vi "Replace Board Pixels.vi"(8 "error in (no error)":errorcluster caption="entrée d'erreur (pas d'erreur)", 9 "New pixels color":u32(colorbox), 10 "Pixels":T1[](array[typedef]), 11 "Game Board en entrée":refnum<class "Game Board.lvclass">) -> (0 "error out":errorcluster caption="sortie d'erreur", 3 "Game Board en sortie":refnum<class "Game Board.lvclass">)   [LabVIEW 2017, in "Game Board.lvclass"]
uses:
  Game Board.lvclass
  Controls/Coordinates.ctl
  Game Board.lvclass/Game Board.ctl
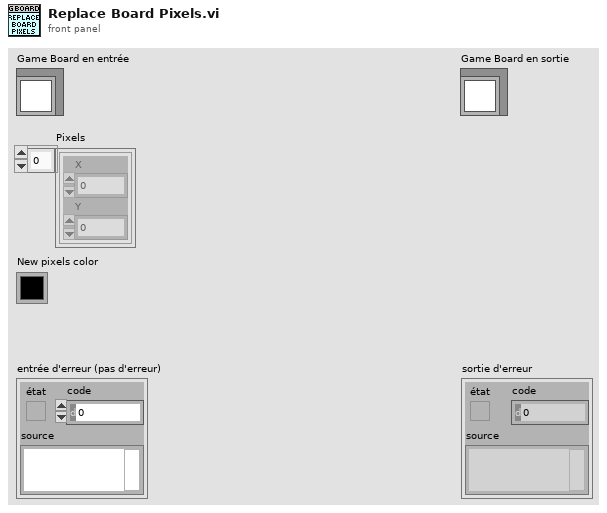
[diagram p1: front panel]
types:
  T1 = typedef "Coordinates.ctl" = cluster{"X":i32, "Y":i32}
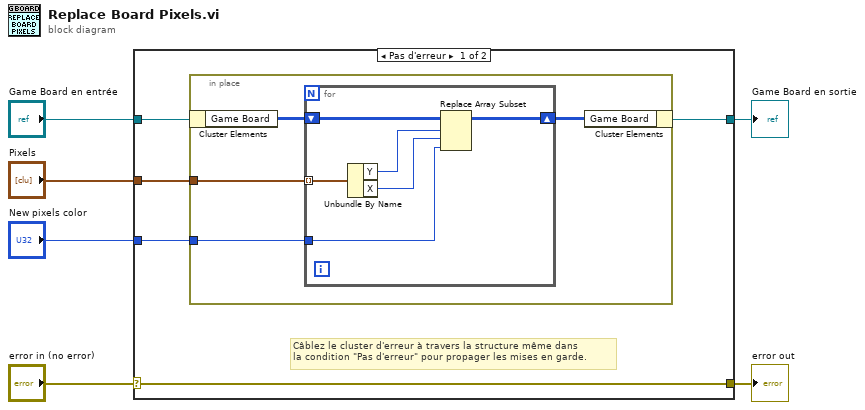
[diagram p0: block diagram]
diagram:
  n1 = case shown="Pas d'erreur" "error in (no error)" {
    selector: "error in (no error)" -> [w11 w23]
    tunnel: [w11 w23] -> w5
    tunnel: [w9 w22] -> w3
    tunnel: "Game Board en entrée" -> [w10 w22]
    tunnel: "Pixels" -> [w8 _]
    tunnel: "New pixels color" -> [w7 _]
    frame No Error {
      # "Câblez le cluster d'erreur à travers la structure même dans\nla condition \"Pas d'erreur\" pour propager les mises en garde."
      n2 = in-place {
        in-place-border: w8 -> [w13]
        in-place-border: w7 -> [w12]
        n3 = in-place-cluster #1(w10) -> ("Game Board"=w15:u32[][])
        n4 = for {
          shift-right: [w20] -> w14
          shift-left: w15 -> [w21]
          tunnel: w13 -> [w19] mode=indexing
          tunnel: w12 -> [w16]
          n5 = Unbundle By Name(w19) -> ("Y"=w18:i32, "X"=w17:i32)
          n6 = Replace Array Subset(array=w21, new element=w16, index (row)=w18, index (col)=w17) -> (w20:u32[][])
        }
        n7 = in-place-cluster #1("Game Board"=w14) -> (w9:refnum<class "Game Board.lvclass">)
      }
    }
    frame Error {
    }
  }
  "error out" <- w5
  "Game Board en sortie" <- w3
